vi "1DTurnMain.vi"() -> ()   [LabVIEW 2017]
panel:
  out "Done?":bool
  out "Vel":cluster{"Output":dbl, "dx/dt":dbl}(graph)={"Output"=47.4353047807108, "dx/dt"=76.52582126109495}
  in  "Gains":T1={"FFV"=0.0032, "FFA"=0.0, "Vel PID"={"P"=0.0, "I"=0.0, "D"=0.0}} {"Vel PID"."D" format="%.3f"; "Vel PID"."I" format="%.3f"; "Vel PID"."P" format="%.3f"}
  out "Pos":dbl(graph)=299.88802132939395
  in  "Config":T2={"Gear Reduction"=15.0, "Wheel Radius (m)"=0.076, "# Motors"=6, "coeff of friction"=0.1, "Mass (kg)"=50.0, "Motor"={"Ke (V)"=0.0183, "R (ohms)"=0.09, "KT (Nm/A)"=0.0183, "Tf (Nm)"=0.4}}
  in  "Distance":dbl=300.0
  in  "MaxVel":dbl=80.0
  in  "MaxAccel":dbl=120.0
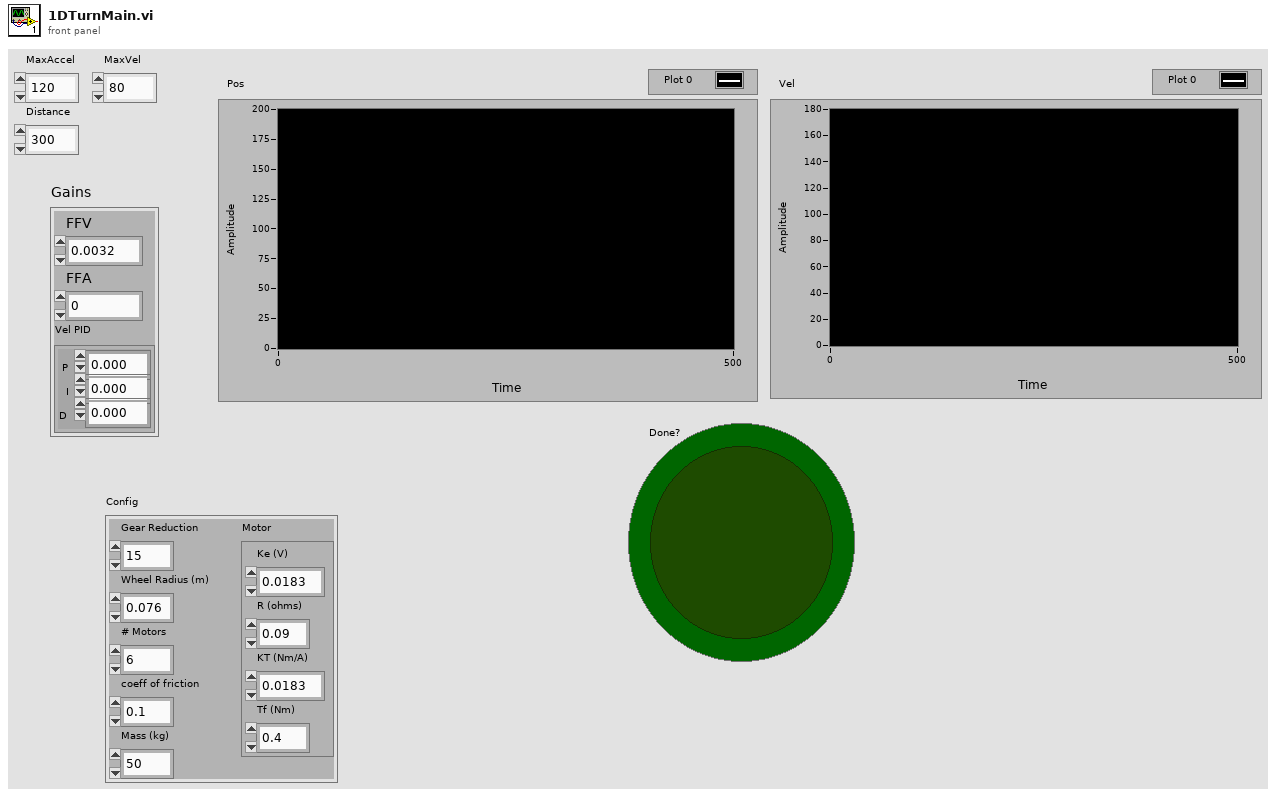
[diagram p1: front panel]
types:
  T1 = cluster{"FFV":dbl, "FFA":dbl, "Vel PID":cluster{"P":dbl, "I":dbl, "D":dbl}}
  T2 = cluster{"Gear Reduction":dbl, "Wheel Radius (m)":dbl, "# Motors":u32, "coeff of friction":dbl, "Mass (kg)":dbl, "Motor":cluster{"Ke (V)":dbl, "R (ohms)":dbl, "KT (Nm/A)":dbl, "Tf (Nm)":dbl}}
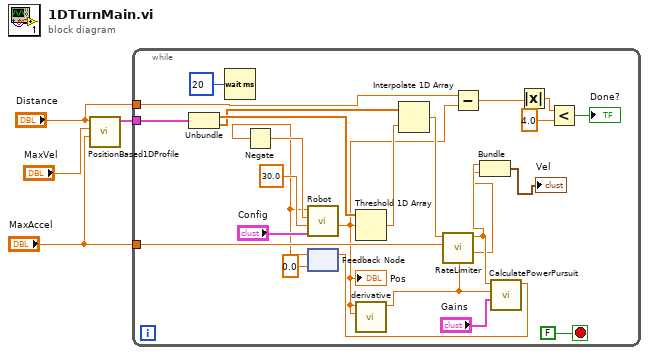
[diagram p0: block diagram]
diagram:
  n1 = call "PositionBased1DProfile.vi"("MaxAccel"="MaxAccel", "MaxVel"="MaxVel", "Distance"="Distance") -> ("Profile"=w3:cluster{"Distances":dbl[], "Vels":dbl[]})  [unwired: 8 in]
  n2 = while {
    tunnel: w3 -> [w27]
    tunnel: "MaxAccel" -> [w20]
    tunnel: "Distance" -> [w11]
    stop <- FALSE stop-if-true
    n3 = Unbundle(w27) -> ("Distances"=w24:dbl[], "Vels"=w23:dbl[])
    n4 = Wait (ms)(milliseconds to wait=u32 20) -> ()  [unwired: 1 out]
    n5 = feedback #1(0.0 ("Power")) -> (w16:dbl)
    n6 = Negate(x=w16) -> (-x=w19:dbl)
    n7 = call "Robot.vi"("Config"="Config", "WheelBase"=30.0, "Right Value"=w19, "Left Value"=w16) -> ("Angle"=w10:dbl)  [unwired: 5 in, 2 out]
    "Pos" <- w10
    n8 = Threshold 1D Array(2:w10, 3:w24) -> (0:w22:dbl)  [unwired: 1 in]
    n9 = call "derivative.vi"("Starting value"=w10, "x"=w10) -> ("dx/dt"=w13:dbl)  [unwired: 9 in]
    n10 = Interpolate 1D Array(1:w22, 2:w23) -> (0:w21:dbl)
    n11 = call "RateLimiter.vi"("Max dx/dt"=w20, "Input"=w21) -> ("Output"=w14:dbl)  [unwired: 9 in]
    n12 = Subtract(x=w11, y=w10) -> (x-y=w9:dbl)
    n13 = Bundle("Output"=w14, "dx/dt"=w13) -> (→"Vel":cluster{"Output":dbl, "dx/dt":dbl})  [unwired: 1 in]
    n14 = call "CalculatePowerPursuit.vi"("Gains"="Gains", "Vel"=w13, "Target Vel"=w14) -> ("Power"=w17:dbl)  [unwired: 8 in]
    n15 = feedback-in #1(w17) -> ()
    n16 = Absolute Value(x=w9) -> (abs(x)=w8:dbl)
    n17 = Less?(x=w8, y=4.0) -> (x < y?=→"Done?":bool)
  }
